vi "Universal Power Meter.vi"() -> ()   [LabVIEW 2013]
uses:
  <vilib>/ActorFramework/Message Queue/Message Queue.lvclass/Message Queue.ctl
  Universal Power Meter.lvclass
  <vilib>/ActorFramework/Message Enqueuer/Message Enqueuer.lvclass/Message Enqueuer.ctl
  <vilib>/ActorFramework/Message Enqueuer/Enqueue.vi
  <vilib>/ActorFramework/Message Priority Queue/Priority Enqueue.vi
  <vilib>/ActorFramework/Stop Msg/Stop Msg.lvclass
  <vilib>/ActorFramework/Message Queue/Message Queue.lvclass
  <vilib>/ActorFramework/Actor/Actor.lvclass
  fileVersionInfo/fileversion.lvlib
panel:
  out "Version":string
  in  "Reset?":bool=TRUE
  out "ID cluster.Model":string
  out "Address":string
  out "error out  (no error)":errorcluster
  in  "Stop Button":bool
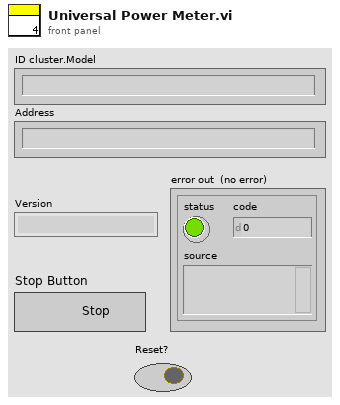
[diagram p1: front panel]
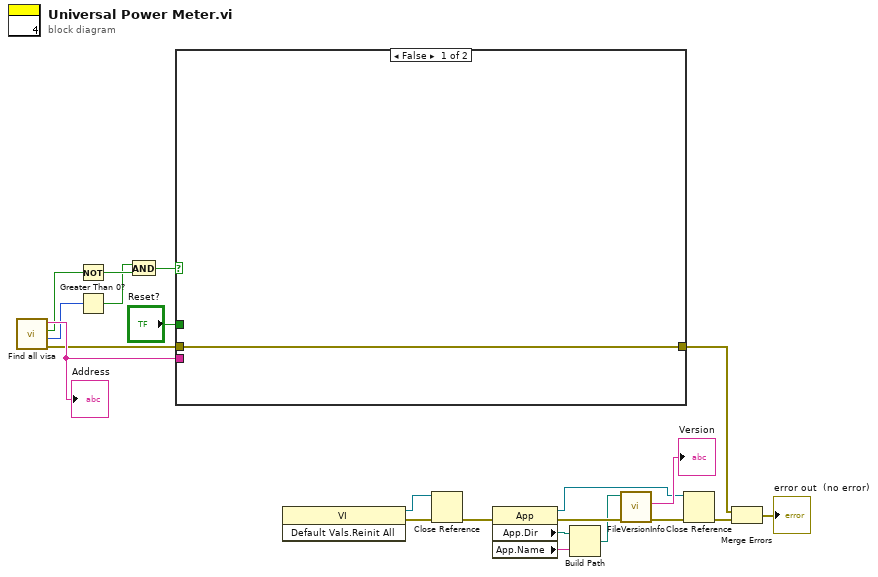
[diagram p0: block diagram]
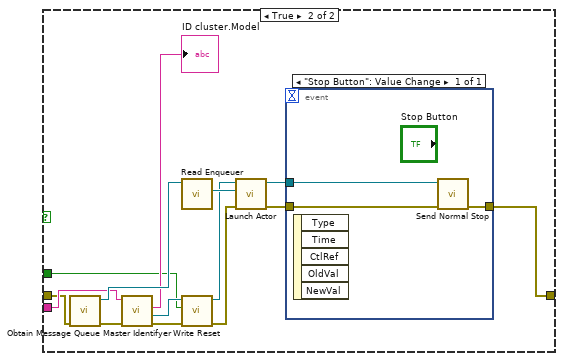
[diagram p2: hidden frame]
diagram:
  n1 = call "Find all visa.vi"() -> ("error out"=w20:errorcluster, "# of Address Found"=w15:i32, "Cancelled?"=w16:bool, "element"=w21:string)  [unwired: 8 in]
  "Address" <- w21
  n2 = Not(x=w16) -> (.not. x?=w19:bool)
  n3 = Greater Than 0?(x=w15) -> (x > 0?=w18:bool)
  n4 = And(x=w18, y=w19) -> (x .and. y?=w17:bool)
  n5 = case shown="False" w17 {
    tunnel: [w22 w31] -> w2
    tunnel: w21 -> [_ w33]
    tunnel: w20 -> [w22 w32]
    tunnel: "Reset?" -> [_ w24]
    frame False {
    }
    frame True {
      n6 = call <vilib>:"Obtain Message Queue.vi"("error in (no error)"=w32) -> ("error out"=w29:errorcluster, "Message Queue"=w36:refnum<class "Message Queue.lvclass">)  [unwired: 9 in]
      n7 = call "Master Identifyer.vi"("error in (no error) 2"=w29, "VISA resource name"=w33) -> ("error out (no error)"=w26:errorcluster, "Class out"=w28:refnum<class "Universal Power Meter.lvclass">, "ID cluster.Model"=→"ID cluster.Model":string)  [unwired: 5 in, 2 out]
      n8 = call <vilib>:"Read Enqueuer.vi"("Message Queue"=w36) -> ("Message Enqueuer"=w35:refnum<class "Message Enqueuer.lvclass">)  [unwired: 10 in]
      n9 = call-dynamic "Write Reset.vi"("error in (no error)"=w26, "Reset"=w24, "Generic Instrument in"=w28) -> ("error out"=w25:errorcluster, "Generic Instrument out"=w27:refnum<class "Universal Power Meter.lvclass">)  [unwired: 7 in]
      n10 = call <vilib>:"Launch Actor.vi"("error in (no error)"=w25, "Actor-to-Caller Enqueuer"=w35, "Actor"=w27) -> ("error out"=w23:errorcluster, "Caller-To-Actor Enqueuer"=w34:refnum<class "Message Enqueuer.lvclass">)  [unwired: 7 in]
      n11 = event shown="[0] \"Stop Button\": Value Change" {
        selector: _ -> [_]
        dyn-events: _ -> [_]
        timeout: _ -> [_]
        tunnel: [w39] -> w31
        tunnel: w34 -> [w38]
        tunnel: w23 -> [w37]
        event "Stop Button": Value Change {
          n12 = event-data() -> ()  [unwired: 1 in, 5 out]
          n13 = call <vilib>:"Send Normal Stop.vi"("error in (no error)"=w37, "Message Enqueuer"=w38) -> ("error out"=w39:errorcluster)  [unwired: 9 in]
        }
      }
    }
  }
  n14 = invoke class="VI" method="Default Vals.Reinit All"() -> (reference out=w9:refnum<vi>, error out=w11:errorcluster)  [unwired: 3 in, 1 out]
  n15 = Close Reference(reference=w9, error in (no error)=w11) -> (error out=w10:errorcluster)
  n16 = property class="App"(error in=w10) -> (reference out=w5:refnum<vi>, error out=w12:errorcluster, "App.Dir"=w8:path, "App.Name"=w7:string)  [unwired: 1 in]
  n17 = Build Path(base path=w8, name or relative path=w7) -> (appended path=w6:path)
  n18 = call "FileVersionInfo.vi"("error in (no error)"=w12, "Application Path in"=w6) -> ("error out"=w4:errorcluster, "File Version Info"=→"Version":string)  [unwired: 6 in, 2 out]
  n19 = Close Reference(reference=w5, error in (no error)=w4) -> (error out=w3:errorcluster)
  n20 = Merge Errors(w2, w3) -> (→"error out  (no error)":errorcluster)
